vi "FinalizeHWI.vi"(8 "error in (no error)":errorcluster, 10 "Master Device in":refnum<class "Master Device.lvclass">, 11 "Device in":refnum<class "Device.lvclass">) -> (0 "error out":errorcluster, 2 "Master Device out":refnum<class "Master Device.lvclass">, 3 "Device out":refnum<class "Device.lvclass">)   [LabVIEW 2013, in "Device.lvclass"]
doc: "FinalizeHWI is run after ALL devices have had a chance to request triggering. So that multiple devices can share a trigger line, each device needs to implement the subVIs called within: \n (1) Prune.vi (look at triggering again and remove lines which do not need to be triggered) and then\n (2) BuildHWI.vi (take pruned \"Prepared\" data and build the HWI in normal time-ordered form to be written to the device in LoadHardware.vi)."
uses:
  Device.lvclass
  Master Device/Master Device.lvclass
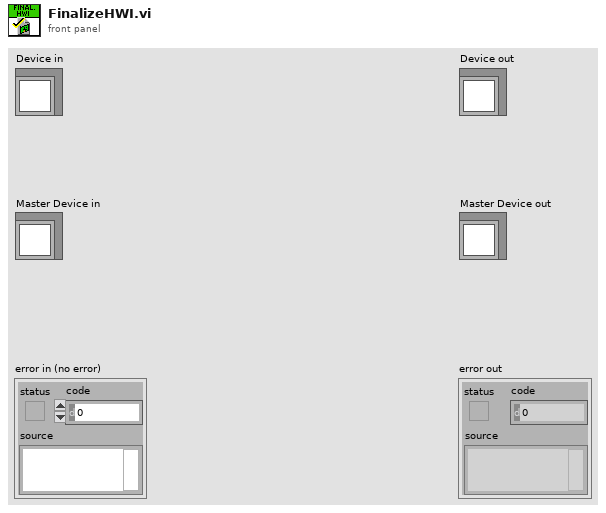
[diagram p1: front panel]
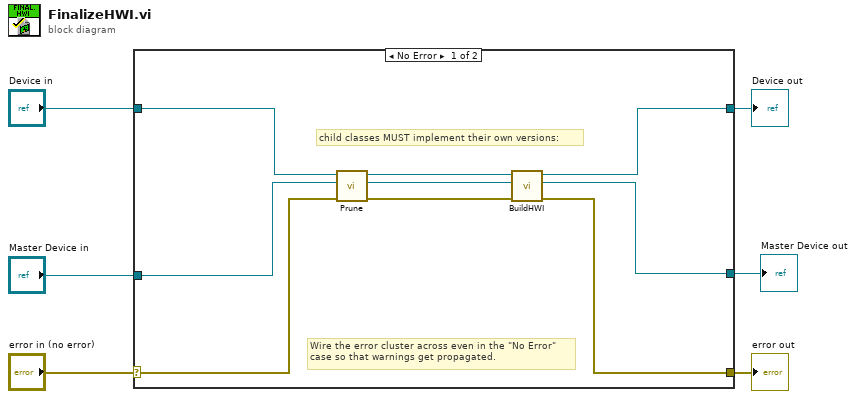
[diagram p0: block diagram]
diagram:
  n1 = case shown="No Error" "error in (no error)" {
    selector: "error in (no error)" -> [w8 w18]
    tunnel: [w7 w18] -> w5
    tunnel: [w13 w17] -> w3
    tunnel: "Device in" -> [w15 w17]
    tunnel: "Master Device in" -> [w12 w16]
    tunnel: [w9 w16] -> w1
    frame No Error {
      # "child classes MUST implement their own versions:"
      # "Wire the error cluster across even in the \"No Error\"\ncase so that warnings get propagated."
      n2 = call-dynamic "Prune.vi"("error in (no error)"=w8, "Master Device in"=w12, "Device in"=w15) -> ("error out"=w10:errorcluster, "Master Device out"=w11:refnum<class "Master Device.lvclass">, "Device out"=w14:refnum<class "Device.lvclass">)  [unwired: 6 in]
      n3 = call-dynamic "BuildHWI.vi"("error in (no error)"=w10, "Master Device in"=w11, "Device in"=w14) -> ("error out"=w7:errorcluster, "Master Device out"=w9:refnum<class "Master Device.lvclass">, "Device out"=w13:refnum<class "Device.lvclass">)  [unwired: 6 in]
    }
    frame Error {
    }
  }
  "error out" <- w5
  "Device out" <- w3
  "Master Device out" <- w1
